vi "getViGetEvent.vi"(8 "error in (no error)":errorcluster, 10 "name":string, 11 "LibReader in":refnum<class "LibReader.lvclass">) -> (0 "error out":errorcluster, 1 "clusterNameOutput":string, 2 "pathViGetEvent":path, 3 "LibReader out":refnum<class "LibReader.lvclass">)   [LabVIEW 2018, in "LibReader.lvclass"]
doc: "Get the path of get event vi."
uses:
  LibReader.lvclass
  LibReader.lvclass/LibReader.ctl
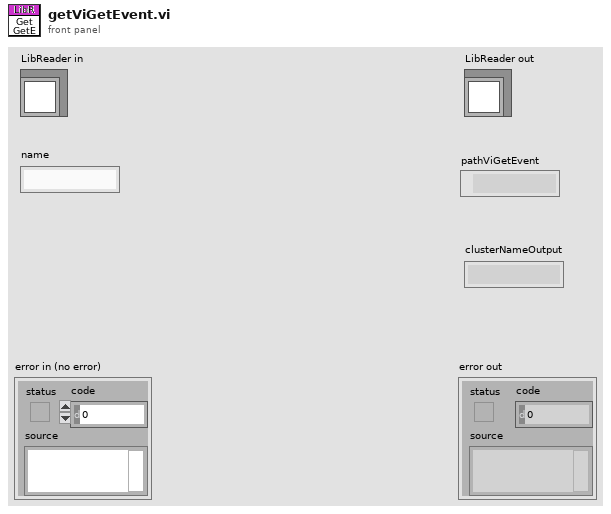
[diagram p1: front panel]
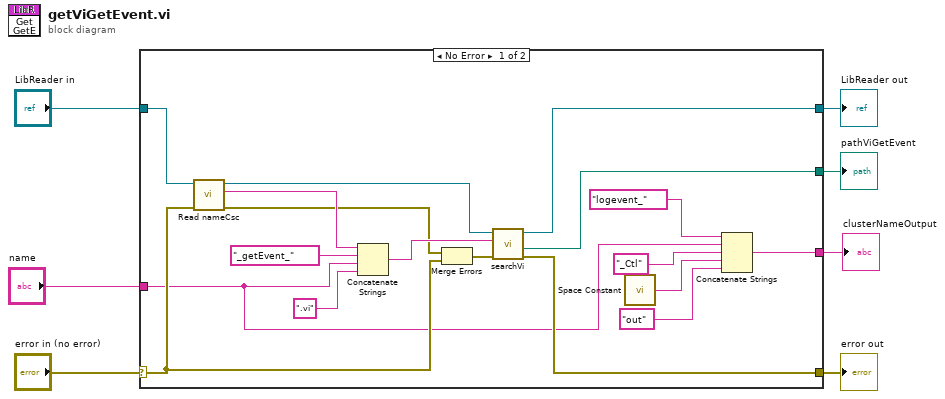
[diagram p0: block diagram]
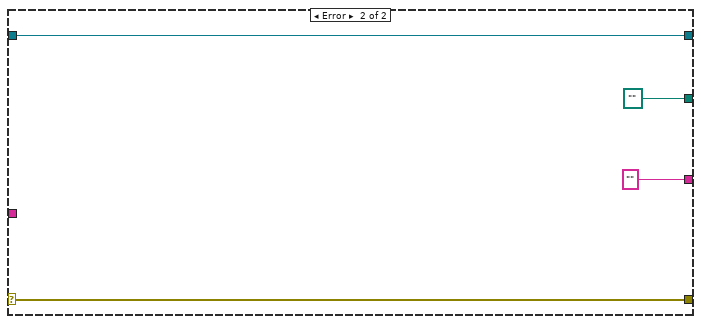
[diagram p2: hidden frame]
diagram:
  n1 = case shown="No Error" "error in (no error)" {
    selector: "error in (no error)" -> [w17 w29]
    tunnel: [w16 w29] -> w6
    tunnel: [w14 w28] -> w4
    tunnel: "LibReader in" -> [w21 w28]
    tunnel: [w25 path "" ("pathVi")] -> w3
    tunnel: "name" -> [w11 _]
    tunnel: [w8 ""] -> w1
    frame No Error {
      n2 = call "Read nameCsc.vi"("error in (no error)"=w17, "LibReader in"=w21) -> ("error out"=w18:errorcluster, "nameCsc"=w20:string, "LibReader out"=w15:refnum<class "LibReader.lvclass">)  [unwired: 7 in]
      n3 = Concatenate Strings(w20, "_getEvent_" ("regExpr"), w11, ".vi" ("regExpr")) -> (w22:string)
      n4 = Merge Errors(w18, w17) -> (w19:errorcluster)
      n5 = call "searchVi.vi"("error in (no error)"=w19, "regExpr"=w22, "LibReader in"=w15) -> ("error out"=w16:errorcluster, "pathVi"=w25:path, "LibReader out"=w14:refnum<class "LibReader.lvclass">)  [unwired: 5 in, 1 out]
      n6 = call <vilib>:"Space Constant.vi"() -> ("String"=w10:string)
      n7 = Concatenate Strings("logevent_", w11, "_Ctl", w10, "out") -> (w8:string)
    }
    frame Error {
    }
  }
  "error out" <- w6
  "LibReader out" <- w4
  "pathViGetEvent" <- w3
  "clusterNameOutput" <- w1
